vi "set_text_color.vi"() -> ()   [LabVIEW 2022 SP3]
panel:
  in  "stop":bool
  in  "Text.Text Colors:Text Color":u32(colorbox)
  out "String":string
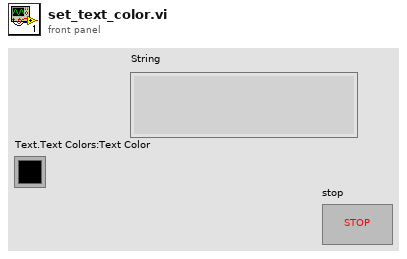
[diagram p1: front panel]
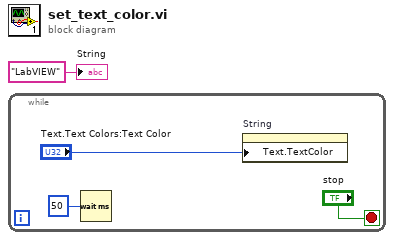
[diagram p0: block diagram]
diagram:
  n1 = while {
    stop <- "stop" stop-if-true
    n2 = Wait (ms)(milliseconds to wait=u32 50) -> ()  [unwired: 1 out]
    n3 = property on="String" class="Str"("Text.TextColor"="Text.Text Colors:Text Color") -> ()  [unwired: 2 in, 2 out]
  }
  "String" <- "LabVIEW" ("String")
